vi "Add Report Section.vi"(6 "Step Number":i32, 7 "Report Path":path, 8 "error in (no error)":errorcluster, 9 "Report Data":T1, 10 "Report in":refnum<class "NI_report.lvclass">, 11 "Image Assertion in":refnum<class "Image Assertion.lvclass">) -> (0 "error out":errorcluster, 2 "Report out":refnum<class "NI_report.lvclass">, 3 "Image Assertion out":refnum<class "Image Assertion.lvclass">)   [LabVIEW 2020, in "MacroAssert.lvlib" / "Image Assertion.lvclass"]
uses:
  Image Assertion.lvclass
  <vilib>/Utility/NIReport.llb/NI_report.lvclass
  Image Assertion.lvclass/Image Assertion.ctl
  <vilib>/picture/picture.llb/imagedata.ctl
  <vilib>/Utility/NIReport.llb/Append Image to Report (path wrap).vi
  <vilib>/Utility/NIReport.llb/Append Report Text (str wrap).vi
  CTLs/Report Data.ctl
  MacroAssert.lvlib
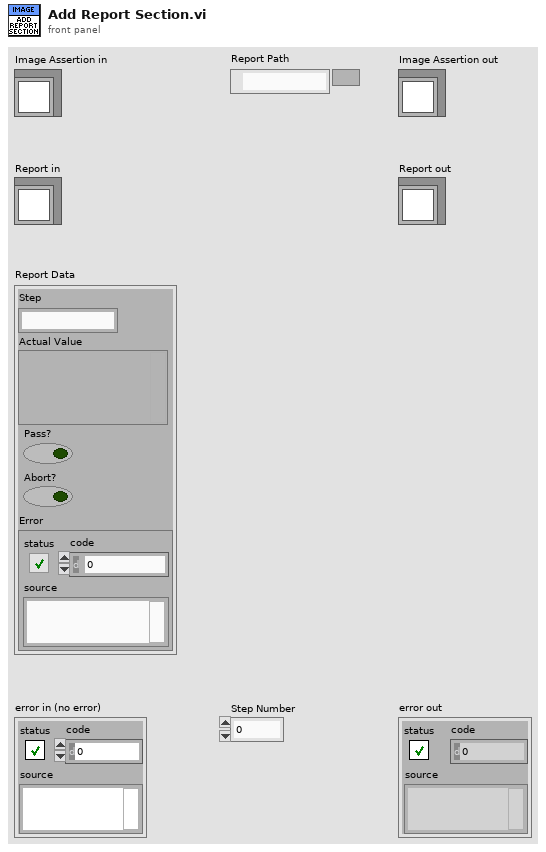
[diagram p1: front panel]
types:
  T1 = typedef "MacroAssert.lvlib/Report Data.ctl" = cluster{"Step":string, "Actual Value":variant, "Pass?":bool, "Abort?":bool, "Error":errorcluster}
  T2 = typedef "imagedata.ctl" = cluster{"image type":i32, "image depth":i32, "image":u8[], "mask":u8[], "colors":u32[], "Rectangle":cluster{"left":i16, "top":i16, "right":i16, "bottom":i16}}
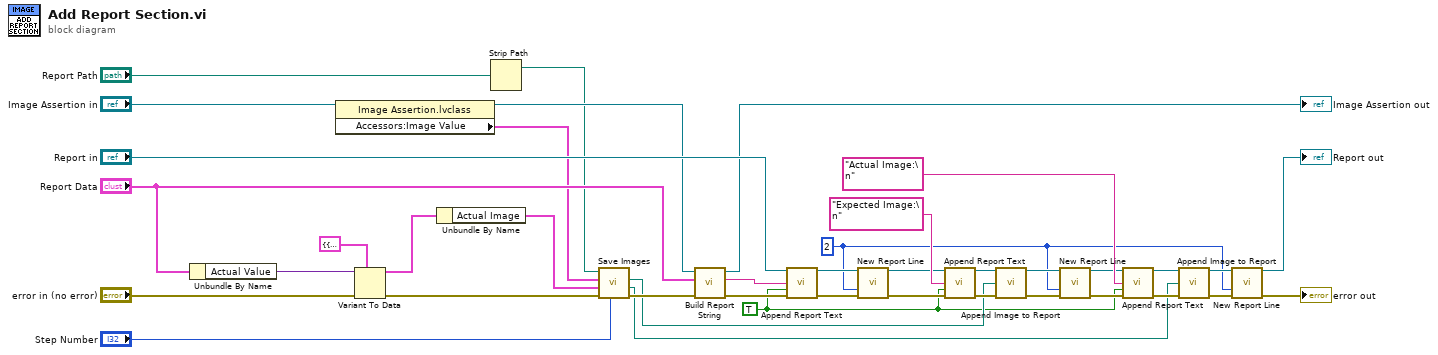
[diagram p0: block diagram]
diagram:
  w1 = 2 ("number of lines (1)")
  w10 = TRUE ("append on new line? (F)")
  n1 = Unbundle By Name("Report Data") -> ("Actual Value"=w25:variant)
  n2 = property class="Image Assertion.lvclass"(reference="Image Assertion in") -> (reference out=w24:refnum<class "Image Assertion.lvclass">, "Accessors:Image Value"=w19:T2)  [unwired: 1 in, 1 out]
  n3 = Variant To Data(error in="error in (no error)", type=cluster{"Actual Image":T2, "Value":dbl} {"Actual Image"={"image type"=0, "image depth"=0, "image"=[], "mask"=[], "colors"=[], "Rectangle"={"left"=0, "top"=0, "right"=0, "bottom"=0}}, "Value"=0.0}, Variant=w25) -> (data=w21:cluster{"Actual Image":T2, "Value":dbl}, error out=w37:errorcluster)
  n4 = Unbundle By Name(w21) -> ("Actual Image"=w18:T2)
  n5 = Strip Path(path="Report Path") -> (stripped path=w17:path)  [unwired: 1 out]
  n6 = call "Save Images.vi"("Step Number"="Step Number", "error in (no error)"=w37, "Actual Image"=w18, "Expected Image"=w19, "Directory"=w17) -> ("error out"=w38:errorcluster, "Actual Image Path"=w15:path, "Expected Image Path"=w14:path)  [unwired: 4 in]
  n7 = call-dynamic "Build Report String.vi"("error in (no error)"=w38, "Report Data"="Report Data", "Image Assertion in"=w24) -> ("error out"=w39:errorcluster, "Report String"=w13:string, "Image Assertion out"=→"Image Assertion out":refnum<class "Image Assertion.lvclass">)  [unwired: 6 in]
  n8 = call-poly <vilib>:"Append Report Text.vi"("report in"="Report in", "text"=w13, "append on new line? (F)"=w10, "error in (no error)"=w39) -> ("report out"=w7:refnum<class "NI_report.lvclass">, "error out"=w34:errorcluster)  [unwired: 8 in, 2 out]
  n9 = call-dynamic "New Report Line.vi"("report in"=w7, "number of lines (1)"=w1, "error in (no error)"=w34) -> ("report out"=w6:refnum<class "NI_report.lvclass">, "error out"=w33:errorcluster)  [unwired: 11 out]
  n10 = call-poly <vilib>:"Append Report Text.vi"("report in"=w6, "text"="Expected Image:\n", "append on new line? (F)"=w10, "error in (no error)"=w33) -> ("report out"=w12:refnum<class "NI_report.lvclass">, "error out"=w36:errorcluster)  [unwired: 8 in, 2 out]
  n11 = call-poly <vilib>:"Append Image to Report.vi"("report in"=w12, "path or URL of image"=w14, "error in (no error)"=w36) -> ("report out"=w4:refnum<class "NI_report.lvclass">, "error out"=w32:errorcluster)  [unwired: 9 in, 2 out]
  n12 = call-dynamic "New Report Line.vi"("report in"=w4, "number of lines (1)"=w1, "error in (no error)"=w32) -> ("report out"=w5:refnum<class "NI_report.lvclass">, "error out"=w31:errorcluster)  [unwired: 11 out]
  n13 = call-poly <vilib>:"Append Report Text.vi"("report in"=w5, "text"="Actual Image:\n", "append on new line? (F)"=w10, "error in (no error)"=w31) -> ("report out"=w9:refnum<class "NI_report.lvclass">, "error out"=w35:errorcluster)  [unwired: 8 in, 2 out]
  n14 = call-poly <vilib>:"Append Image to Report.vi"("report in"=w9, "path or URL of image"=w15, "error in (no error)"=w35) -> ("report out"=w3:refnum<class "NI_report.lvclass">, "error out"=w30:errorcluster)  [unwired: 9 in, 2 out]
  n15 = call-dynamic "New Report Line.vi"("report in"=w3, "number of lines (1)"=w1, "error in (no error)"=w30) -> ("report out"=→"Report out":refnum<class "NI_report.lvclass">, "error out"=→"error out":errorcluster)  [unwired: 11 out]
